vi "Config.vi"(8 "error in (no error)":errorcluster, 10 "Setting":variant, 11 "NI Thermo in":refnum<class "NI Thermo.lvclass">) -> (0 "error out":errorcluster, 3 "NI Thermo out":refnum<class "NI Thermo.lvclass">)   [LabVIEW 2025, in "Thermo.lvlib" / "NI Thermo.lvclass"]
uses:
  NI Thermo.lvclass
  C:/Working copy/tss/Plugin/Engines/Thermo/Thermo Instrument/Thermo Instrument.lvclass
  Thermo configuration/Thermo configuration.lvclass
  NI Thermo.lvclass/NI Thermo.ctl
  Thermo configuration/Thermo configuration.lvclass/Thermo configuration.ctl
  Thermo configuration/Read Thermo Setting.vi
  <vilib>/DAQmx/configure/timing.llb/DAQmx Timing (Sample Clock).vi
  Users/Public/Documents/Sandia National Labs/TSS Plugin/CEF.lvlibp/serializable configuration/CEF_serializable configuration.lvclass
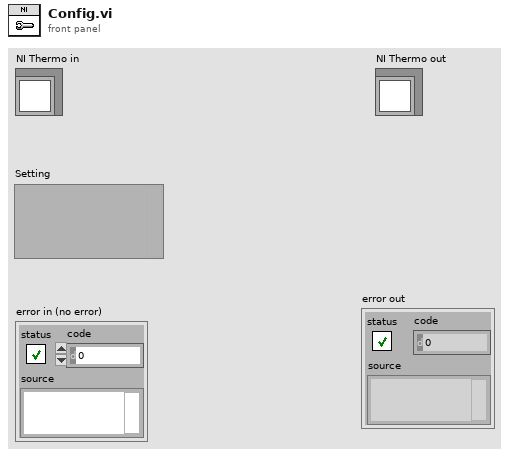
[diagram p1: front panel]
types:
  T1 = typedef "Thermo.lvlib/Thermo configuration.lvclass/Thermo Setting.ctl" = cluster{"Numeric":dbl, "Combo":string, "String":string, "Boolean":bool}
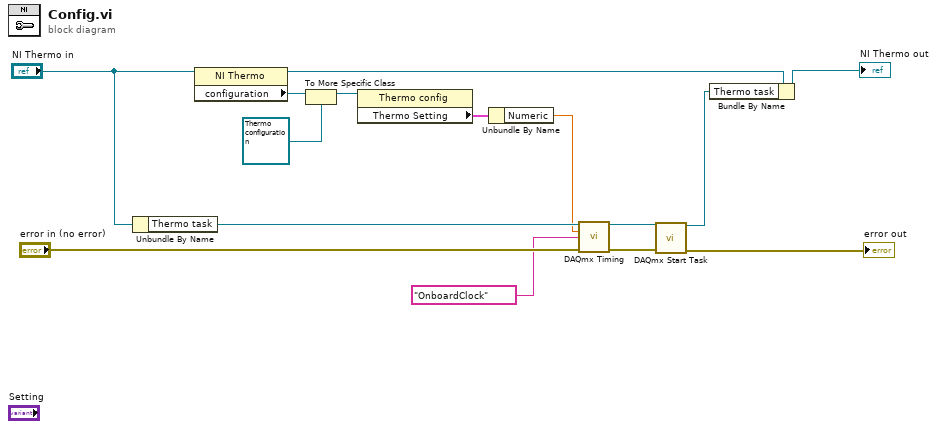
[diagram p0: block diagram]
diagram:
  n1 = Unbundle By Name("NI Thermo in") -> ("Thermo task"=w4:refnum<k21>)
  n2 = property class="NI Thermo"(reference="NI Thermo in") -> (reference out=w12:refnum<class "NI Thermo.lvclass">, "configuration"=w13:refnum<class "CEF_serializable configuration.lvclass">)  [unwired: 1 in, 1 out]
  n3 = To More Specific Class(target class=refnum<class "Thermo configuration.lvclass"> refnum ("DMM.lvlib:DMM configuration.lvclass"), reference=w13) -> (specific class reference=w14:refnum<class "Thermo configuration.lvclass">)  [unwired: 1 in, 1 out]
  n4 = property class="Thermo config"(reference=w14) -> ("Thermo Setting"=w1:T1)  [unwired: 1 in, 2 out]
  n5 = Unbundle By Name(w1) -> ("Numeric"=w3:dbl)
  n6 = call-poly <vilib>:"DAQmx Timing.vi"("task/channels in"=w4, "rate"=w3, "source"=tag "OnboardClock", "error in"="error in (no error)") -> ("task out"=w6:refnum<k21>, "error out"=w7:errorcluster)  [unwired: 10 in]
  n7 = call <vilib>:"DAQmx Start Task.vi"("task/channels in"=w6, "error in"=w7) -> ("task out"=w9:refnum<k21>, "error out"=→"error out":errorcluster)  [unwired: 12 in]
  n8 = Bundle By Name(cluster=w12, "Thermo task"=w9) -> (→"NI Thermo out":refnum<class "NI Thermo.lvclass">)
